vi "digBaseband.vi"() -> ()   [LabVIEW 2013]
uses:
  <vilib>/Analysis/2dsp.llb/1D Convolution (DBL).vi
  <vilib>/Analysis/2dsp.llb/Decimate (single shot, DBL).vi
  <vilib>/Analysis/2dsp.llb/Upsample (DBL).vi
  <vilib>/Analysis/NI_AALPro.lvlib
  <vilib>/Analysis/NI_AALBase.lvlib
panel:
  out "Waveform Graph":dbl[][](graph)
  in  "Enum":enum16{"Sinc", ""}(ring)
  in  "Bit":i32[](array[numeric])
  out "Recovered Bit":i32[](array[numeric])
  out "Symbol":dbl[](array[numeric])
  out "Base band":dbl[](graph)
  in  "sinc samples":i32
  in  "stop":bool
  in  "Up sample factor":i32(slide) scale=0.0..100.0
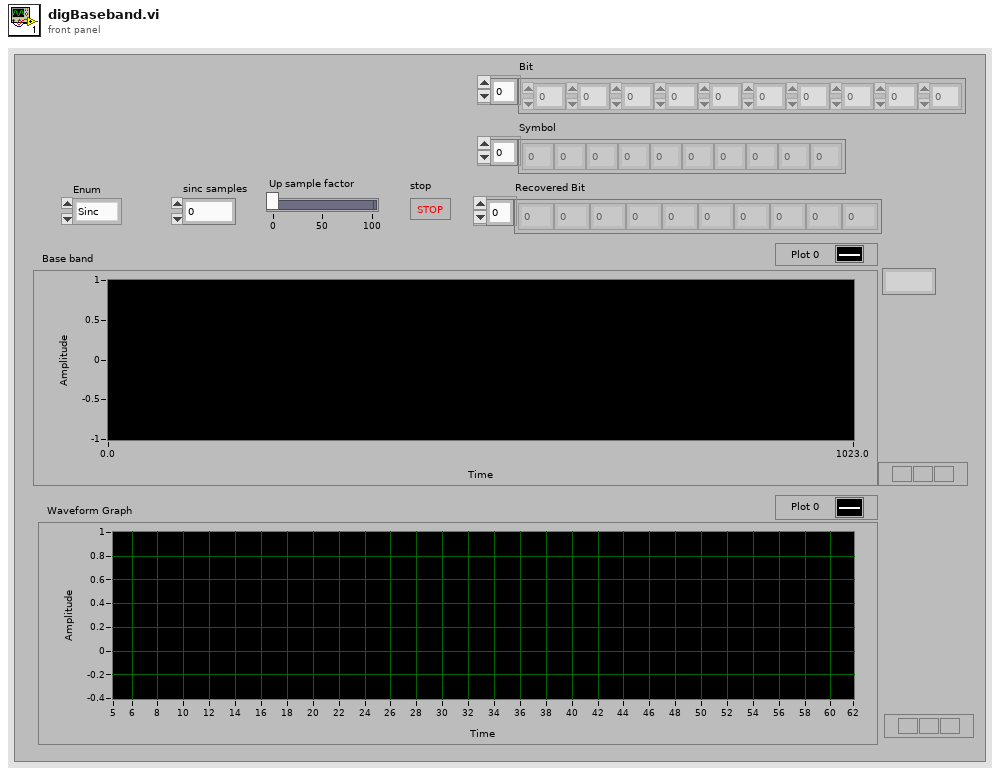
[diagram p1: front panel]
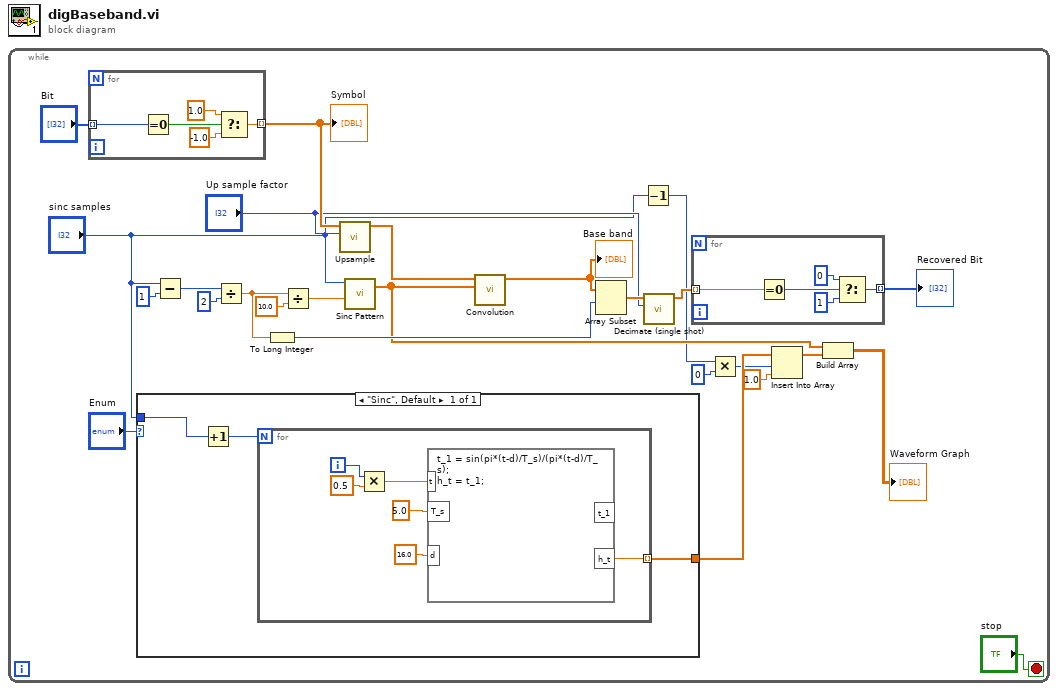
[diagram p0: block diagram]
diagram:
  n1 = while {
    stop <- "stop" stop-if-true
    n2 = for {
      tunnel: [w42] -> w17 mode=indexing
      tunnel: "Bit" -> [w41] mode=indexing
      n3 = Equal To 0?(x=w41) -> (x = 0?=w45:bool)
      n4 = Select(t=1.0, s=w45, f=-1.0) -> (s? t:f=w42:dbl)
    }
    "Symbol" <- w17
    n5 = case shown="\"Sinc\", Default" "Enum" {
      tunnel: "sinc samples" -> [w27]
      tunnel: [w28] -> w9
      frame "Sinc", Default {
        n6 = Increment(x=w27) -> (x+1=w29:i32)
        n7 = for {
          N: w29 -> [_]
          tunnel: [w30] -> w28 mode=indexing
          i -> [w35]
          n8 = Multiply(x=w35, y=0.5) -> (x*y=w33:dbl)
          n9 = formula code="t_1 = sin(pi*(t-d)/T_s)/(pi*(t-d)/T_s);\nh_t = t_1;"("t"=w33, "T_s"=5.0, "d"=16.0) -> ("h_t"=w30:dbl)  [unwired: 1 out]
        }
      }
    }
    n10 = Subtract(x="sinc samples", y=1) -> (x-y=w24:i32)
    n11 = Divide(x=w24, y=2) -> (x/y=w20:dbl)
    n12 = To Long Integer(number=w20) -> (32bit integer=w21:i32)
    n13 = Divide(x=w20, y=10.0) -> (x/y=w11:dbl)
    n14 = call-poly <vilib>:"Upsample.vi"("upsampling factor"="Up sample factor", "X"=w17) -> ("Upsampled Array"=w15:dbl[])  [unwired: 8 in, 1 out]
    n15 = call <vilib>:"Sinc Pattern.vi"("delay"=w11, "samples"="sinc samples") -> ("Sinc Pattern"=w6:dbl[])  [unwired: 2 in, 1 out]
    n16 = call-poly <vilib>:"Convolution.vi"("Y"=w6, "X"=w15) -> ("X * Y"=w13:dbl[])  [unwired: 8 in, 1 out]
    "Base band" <- w13
    n17 = Array Subset(array=w13, index=w21) -> (w26:dbl[])  [unwired: 1 in]
    n18 = Decrement(x="sinc samples") -> (x-1=w5:i32)
    n19 = call-poly <vilib>:"Decimate (single shot).vi"("decimating factor"="Up sample factor", "X"=w26) -> ("Decimated Array"=w14:dbl[])  [unwired: 8 in, 1 out]
    n20 = for {
      tunnel: w14 -> [w37] mode=indexing
      tunnel: [w36] -> w12 mode=indexing
      n21 = Equal To 0?(x=w37) -> (x = 0?=w40:bool)
      n22 = Select(t=0, s=w40, f=1) -> (s? t:f=w36:i32)
    }
    "Recovered Bit" <- w12
    n23 = Multiply(x=w5, y=0) -> (x*y=w3:i32)
    n24 = Insert Into Array(array=w9, index=w3, new element=1.0) -> (w7:dbl[])
    n25 = Build Array(w6, w7) -> (→"Waveform Graph":dbl[][])
  }
